vi "Read EEPROM data file.vi"(8 "error in (no error)":errorcluster, 10 "client ptr":u32, 11 "Estyx device name":string) -> (0 "error out":errorcluster, 2 "Read Data":T1)   [LabVIEW 2010, in "lib1299.lvlib"]
doc: "This VI reads the contents of the EEPROM located on the device EVM (daughtercard).\n\nInputs:\nclient ptr - estyx client pointer to file system\nestyx device name - estyx directory name of the device\nTest mode (debug) - allow for testing without EEPROM input. User must supply string to parse.\n\nOutputs:\nRead Data - cluster of information read from the EEPROM\n - Raw Data: contents of eepage 1 date file from estyx\n - Parsed Data: Raw Data parsed based on memory range for the data value (defined on wiki page for EEPROM information)\n - Data - String: EEPROM data derived from finding the string terminator for each of the Parse Data lines"
uses:
  lib1299.lvlib
  Styx/lvstyx/Write/lvstyx_write_path_int.vi
  Styx/lvstyx/Read/lvstyx_read_all_path.vi
panel:
  in  "Test string":string="4144533132373845564D00FFFFFFFFFFFFFFFFFFFFFFFFFFFFFFFFFFFFFFFFFF363434343039372D5200FFFFFFFFFFFF363434343039382D5500FFFFFFFFFFFF363434343039392D4E00FFFFFFFFFFFF323030383033313900FFFFFFFFFFFFFF"
  in  "Test mode":bool
  # "Test mode:\nTRUE allows user to input text in the \"Text string\" control box\nrather than reading from the estyx file system"
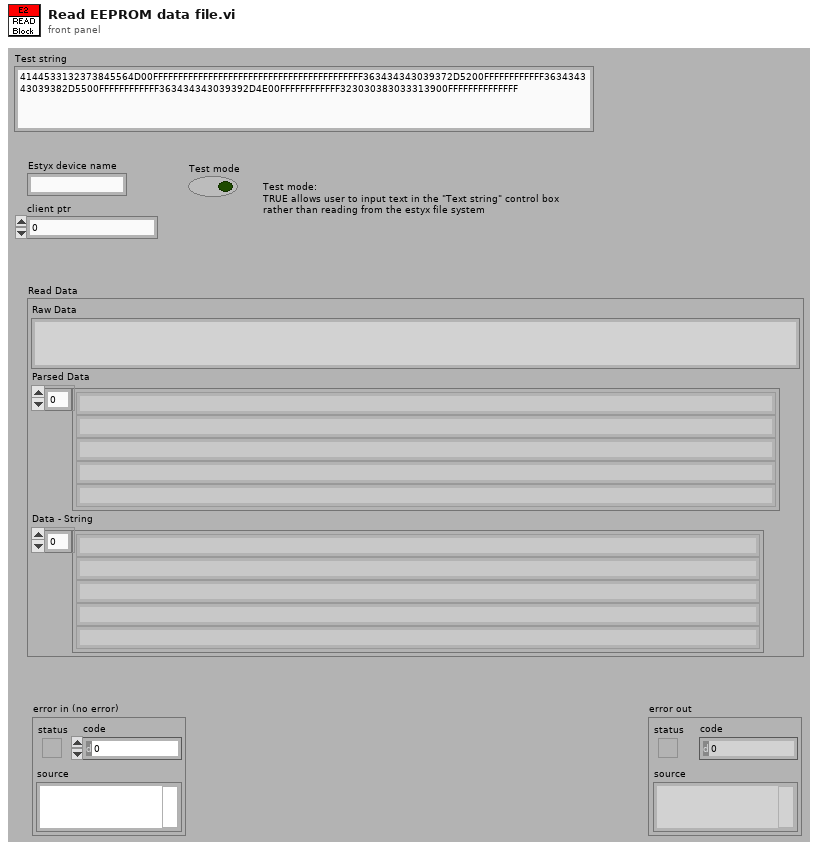
[diagram p1: front panel]
types:
  T1 = typedef "lib1299.lvlib/Read RAW data.ctl" = cluster{"Raw Data":string, "Parsed Data":string[], "Data - String":string[]}
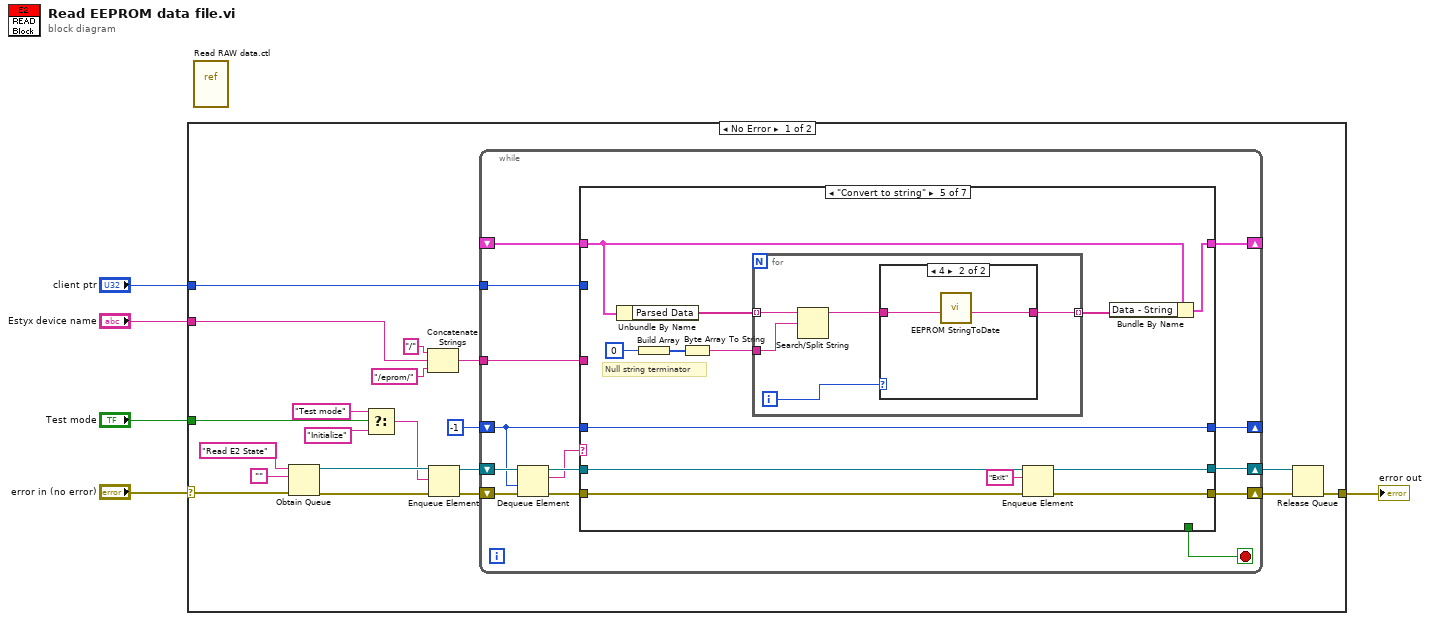
[diagram p0: block diagram]
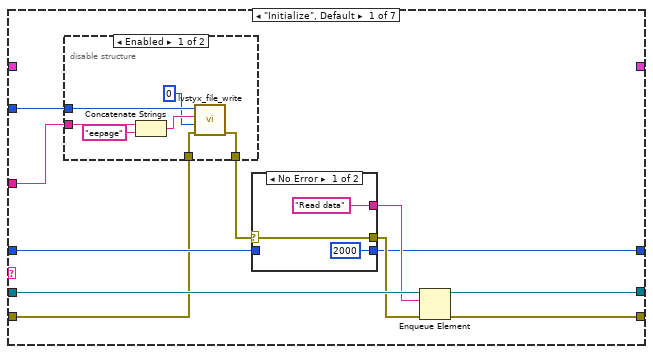
[diagram p2: hidden frame]
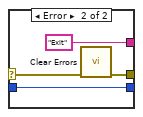
[diagram p4: hidden frame]
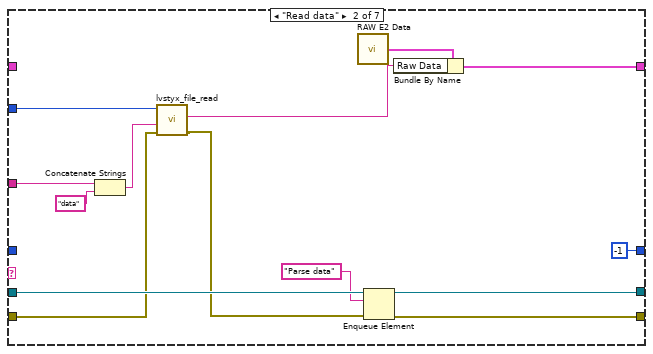
[diagram p5: hidden frame]
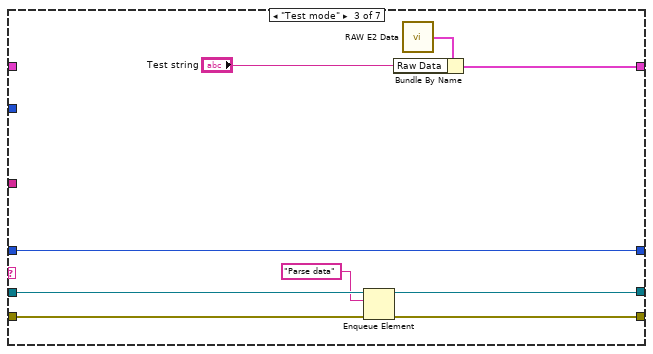
[diagram p6: hidden frame]
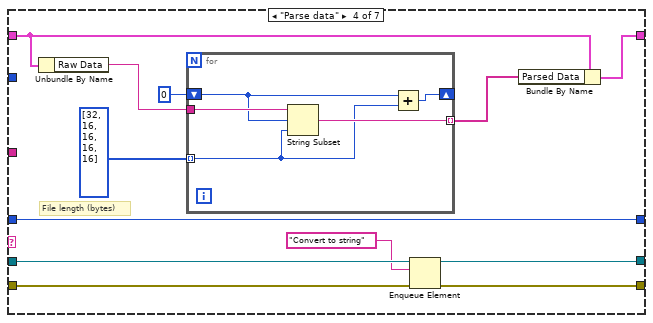
[diagram p7: hidden frame]
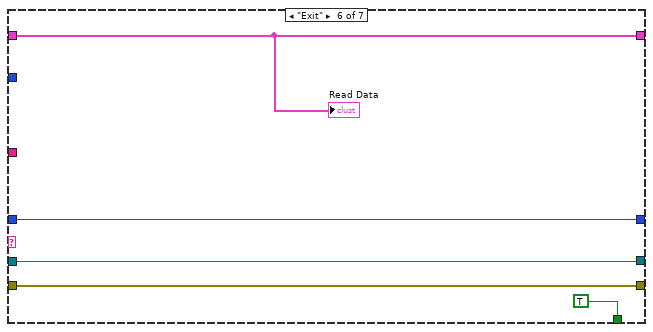
[diagram p9: hidden frame]
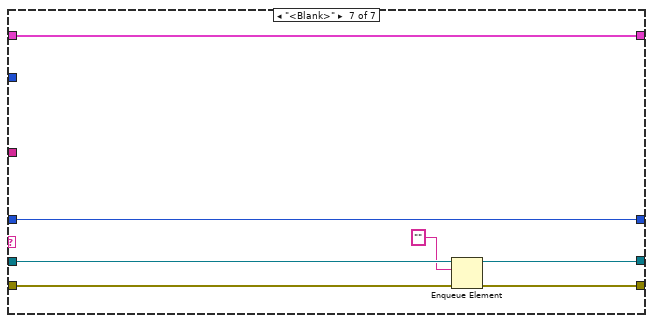
[diagram p10: hidden frame]
diagram:
  n1 = case shown="No Error" "error in (no error)" {
    selector: "error in (no error)" -> [w6 w139]
    tunnel: "Estyx device name" -> [w23 _]
    tunnel: "client ptr" -> [w16 _]
    tunnel: "Test mode" -> [w9 _]
    tunnel: [w7 w139] -> w2
    frame No Error {
      n2 = Obtain Queue(name (unnamed)="Read E2 State", element data type="", error in (no error)=w6) -> (queue out=w20:refnum<queue>, error out=w19:errorcluster)  [unwired: 2 in, 1 out]
      n3 = Select(t="Test mode", s=w9, f="Initialize" ("element")) -> (s? t:f=w11:string)
      n4 = Concatenate Strings("/" ("string"), w23, "/eprom/" ("string")) -> (w15:string)
      n5 = Enqueue Element(queue=w20, element=w11, error in (no error)=w19) -> (queue out=w18:refnum<queue>, error out=w17:errorcluster)  [unwired: 1 in, 1 out]
      n6 = while {
        shift-right: [w35] -> w13
        shift-left: w17 -> [w38]
        shift-right: [w29] -> w12
        shift-left: w18 -> [w39]
        tunnel: w16 -> [w33]
        tunnel: w15 -> [w32]
        shift-right: [w30] -> _
        shift-left: -1 -> [w31]
        shift-right: [w28] -> _
        shift-left: _ -> [w27]
        stop <- w26 stop-if-true
        n7 = Dequeue Element(queue=w39, timeout in ms (-1)=w31, error in (no error)=w38) -> (queue out=w37:refnum<queue>, element=w34:string, error out=w36:errorcluster)  [unwired: 1 out]
        n8 = case shown="\"Convert to string\"" w34 {
          tunnel: w37 -> [w49 w75 w85 w98 w116 w130 w136]
          tunnel: w36 -> [w41 w69 w81 w99 w118 w129 w138]
          tunnel: [w46 w77 w87 w100 w117 w129 w137] -> w35
          tunnel: w33 -> [w42 w70 _ _ _ _ _]
          tunnel: w32 -> [w50 w78 _ _ _ _ _]
          tunnel: w31 -> [w45 _ w88 w94 w111 w131 w133]
          tunnel: [w44 -1 w88 w94 w111 w131 w133] -> w30
          tunnel: [w43 w76 w86 w97 w109 w130 w134] -> w29
          tunnel: [_ w72 w82 w93 w112 w127 w132] -> w28
          tunnel: w27 -> [_ _ _ w92 w113 w127 w132]
          tunnel: [_ _ _ _ _ TRUE _] -> w26
          frame "Initialize", Default {
            n9 = disable-structure shown="Enabled" {
              disable-tunnel: w50 -> [w57 _]
              disable-tunnel: w42 -> [w55 _]
              disable-tunnel: w41 -> [w52 w58]
              disable-tunnel: [w51 w58] -> w40
              frame Enabled {
                n10 = Concatenate Strings(w57, "eepage" ("string")) -> (w54:string)
                n11 = call-poly "lvstyx_file_write.vi"("error in (no error)"=w52, "int64"=i64 0, "path"=w54, "client ptr"=w55) -> ("error out"=w51:errorcluster)  [unwired: 6 in, 1 out]
              }
              frame Disabled {
              }
            }
            n12 = case shown="No Error" w40 {
              selector: w40 -> [w60 w64]
              tunnel: ["Read data" ("element") "Exit" ("element")] -> w47
              tunnel: [w60 w63] -> w48
              tunnel: w45 -> [_ w62]
              tunnel: [2000 w62] -> w44
              frame No Error {
              }
              frame Error {
                n13 = call <vilib>:"Clear Errors.vi"("error in (no error)"=w64) -> ("error out"=w63:errorcluster)  [unwired: 6 in]
              }
            }
            n14 = Enqueue Element(queue=w49, element=w47, error in (no error)=w48) -> (queue out=w43:refnum<queue>, error out=w46:errorcluster)  [unwired: 1 in, 1 out]
          }
          frame "Read data" {
            n15 = Concatenate Strings(w78, "data" ("string")) -> (w66:string)
            n16 = call-poly "lvstyx_file_read.vi"("error in (no error)"=w69, "path"=w66, "client ptr"=w70) -> ("error out"=w68:errorcluster, "buf"=w67:string)  [unwired: 6 in, 1 out]
            n17 = call "RAW E2 Data.vi"() -> ("Read Data"=w73:T1)  [unwired: 1 in]
            n18 = Enqueue Element(queue=w75, element="Parse data", error in (no error)=w68) -> (queue out=w76:refnum<queue>, error out=w77:errorcluster)  [unwired: 1 in, 1 out]
            n19 = Bundle By Name(cluster=w73, "Raw Data"=w67) -> (w72:T1)
          }
          frame "Test mode" {
            n20 = Enqueue Element(queue=w85, element="Parse data", error in (no error)=w81) -> (queue out=w86:refnum<queue>, error out=w87:errorcluster)  [unwired: 1 in, 1 out]
            n21 = call "RAW E2 Data.vi"() -> ("Read Data"=w83:T1)  [unwired: 1 in]
            n22 = Bundle By Name(cluster=w83, "Raw Data"="Test string") -> (w82:T1)
          }
          frame "Parse data" {
            # "File length (bytes)"
            n23 = Unbundle By Name(w92) -> ("Raw Data"=w91:string)
            n24 = for {
              tunnel: i32[] [32, 16, 16, 16, 16] -> [w101] mode=indexing
              shift-right: [w103] -> _
              shift-left: u32 0 -> [w102]
              tunnel: [w104] -> w89 mode=indexing
              tunnel: w91 -> [w105]
              n25 = String Subset(string=w105, offset (0)=w102, length (rest)=w101) -> (substring=w104:string)
              n26 = Add(x=w102, y=w101) -> (x+y=w103:u32)
            }
            n27 = Enqueue Element(queue=w98, element="Convert to string", error in (no error)=w99) -> (queue out=w97:refnum<queue>, error out=w100:errorcluster)  [unwired: 1 in, 1 out]
            n28 = Bundle By Name(cluster=w92, "Parsed Data"=w89) -> (w93:T1)
          }
          frame "Convert to string" {
            # "Null string terminator"
            n29 = Unbundle By Name(w113) -> ("Parsed Data"=w115:string[])
            n30 = Build Array(u8 0) -> (w108:u8[])
            n31 = Byte Array To String(unsigned byte array=w108) -> (string=w106:string)
            n32 = for {
              tunnel: w115 -> [w123] mode=indexing
              tunnel: [w120] -> w114 mode=indexing
              tunnel: w106 -> [w122]
              i -> [w121]
              n33 = Search/Split String(string=w123, search string/char (-)=w122) -> (substring before match=w119:string)  [unwired: 1 in, 2 out]
              n34 = case shown="4" w121 {
                tunnel: [w124 w125] -> w120
                tunnel: w119 -> [w124 w126]
                frame Default {
                }
                frame 4 {
                  n35 = call "EEPROM StringToDate.vi"("Date String"=w126) -> ("Date"=w125:string)  [unwired: 9 in, 1 out]
                }
              }
            }
            n36 = Enqueue Element(queue=w116, element="Exit", error in (no error)=w118) -> (queue out=w109:refnum<queue>, error out=w117:errorcluster)  [unwired: 1 in, 1 out]
            n37 = Bundle By Name(cluster=w113, "Data - String"=w114) -> (w112:T1)
          }
          frame "Exit" {
            "Read Data" <- w127
          }
          frame "<Blank>" {
            n38 = Enqueue Element(queue=w136, element="", error in (no error)=w138) -> (queue out=w134:refnum<queue>, error out=w137:errorcluster)  [unwired: 1 in, 1 out]
          }
        }
      }
      n39 = Release Queue(queue=w12, error in (no error)=w13) -> (error out=w7:errorcluster)  [unwired: 1 in, 2 out]
    }
    frame Error {
    }
  }
  "error out" <- w2
  n40 = vi-ref "Read RAW data.ctl"() -> ()  [unwired: 1 out]
